vi "Insert Conditional.vi"(0 "Test Executive Ref":refnum<data-value>, 1 "Name":string, 2 "Unique ID":string, 3 "Insertion Index":i32=-1, 4 "Assertion":refnum<class "Assert.lvclass">, 5 "error in (no error)":errorcluster, 6 "Parent ID":string, 7 "Variable X":string, 9 "Variable Y":string, 11 "Passing Executive":string, 13 "Failing Executive":string) -> (12 "Unique ID out":string, 14 "Test Executive Ref out":refnum<data-value>, 17 "Replaced?":bool, 19 "error out":errorcluster)   [LabVIEW 2020, in "Test Executive.lvlib" / "TestExecutive Ref.lvclass"]
uses:
  <vilib>/gpm_packages/@cs/test-executive/Source/Test Executive/TestExecutive Ref/TestExecutive Ref.lvclass
  <vilib>/gpm_packages/@cs/test-executive/Source/Test Executive/ITestExecutive/ITest Executive.lvclass
  <vilib>/gpm_packages/@cs/run-time-assertions/Source/Assert/Assert.lvclass
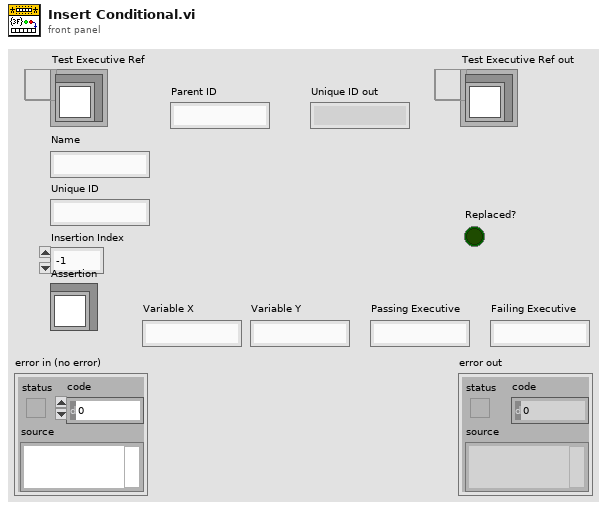
[diagram p1: front panel]
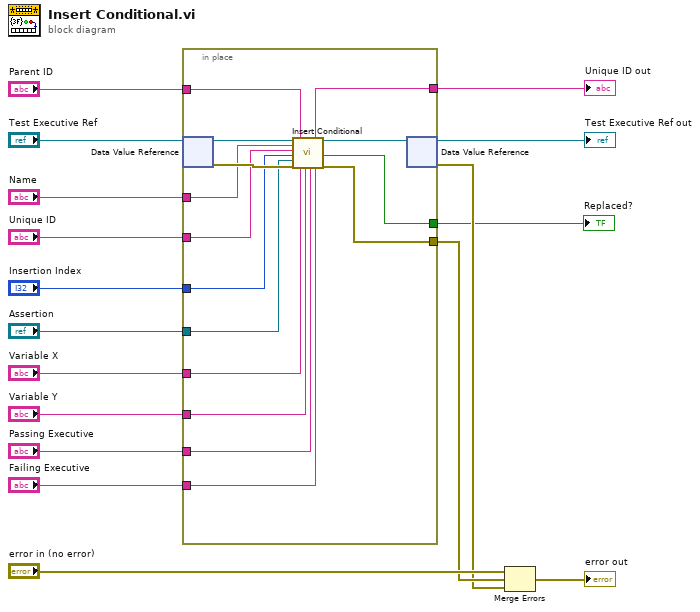
[diagram p0: block diagram]
diagram:
  n1 = in-place {
    in-place-border: "Parent ID" -> [w30]
    in-place-border: "Name" -> [w26]
    in-place-border: "Unique ID" -> [w25]
    in-place-border: "Insertion Index" -> [w24]
    in-place-border: [w29] -> w12
    in-place-border: [w27] -> w10
    in-place-border: "Assertion" -> [w23]
    in-place-border: "Variable X" -> [w22]
    in-place-border: "Variable Y" -> [w21]
    in-place-border: "Passing Executive" -> [w20]
    in-place-border: "Failing Executive" -> [w19]
    in-place-border: [w18] -> w1
    n2 = in-place-dvr #1("Test Executive Ref") -> (w32:refnum<class "ITest Executive.lvclass">, w28:errorcluster)
    n3 = call-dynamic "Insert Conditional.vi"("ITest Executive in"=w32, "Name"=w26, "Unique ID"=w25, "Insertion Index"=w24, "Assertion"=w23, "error in (no error)"=w28, "Parent ID"=w30, "Variable X"=w22, "Variable Y"=w21, "Passing Executive"=w20, "Failing Executive"=w19) -> ("Unique ID out"=w29:string, "ITest Executive out"=w31:refnum<class "ITest Executive.lvclass">, "Replaced?"=w18:bool, "error out"=w27:errorcluster)  [unwired: 5 in]
    n4 = in-place-dvr #1(w31) -> (→"Test Executive Ref out":refnum<data-value>, w9:errorcluster)
  }
  "Unique ID out" <- w12
  "Replaced?" <- w1
  n5 = Merge Errors("error in (no error)", w10, w9) -> (→"error out":errorcluster)
